vi "Configure.vi"(8 "error in (no error)":errorcluster, 11 "Measurement in":refnum<class "Measurement.lvclass">) -> (0 "error out":errorcluster, 3 "Measurement out":refnum<class "Measurement.lvclass">)   [LabVIEW 2017, in "Measurement Actor.lvlib" / "Measurement.lvclass"]
doc: "Override configure.vi to setup any parameters for a measurement before acquiring.\n\nConfigure.vi is called by the 'Initialize Measurement Actor Core.vi,' which executes before Actor Core of the root measurement class. The root configure method populates the basic Measurement UI with information such as the hardware device in use and the name of the measurement. The base configure method calls 'Acquire.vi' once execution is complete. If beginning a recurring acquisition, it reset the iteration count to zero."
uses:
  Measurement.lvclass
  C:/Program Files (x86)/National Instruments/LabVIEW 2017/vi.lib/ActorFramework/Actor/Actor.lvclass
  <vilib>/ActorFramework/Actor/Actor.lvclass/Actor.ctl
  <vilib>/ActorFramework/Message Enqueuer/Message Enqueuer.lvclass/Message Enqueuer.ctl
  Hardware/Hardware.lvclass/Hardware.ctl
  <vilib>/ActorFramework/Message Enqueuer/Init from Existing Queue.vi
  <vilib>/ActorFramework/Message Enqueuer/Enqueue.vi
  Messages/Acquire Msg/Acquire Msg.lvclass
  C:/Program Files (x86)/National Instruments/LabVIEW 2017/vi.lib/ActorFramework/Message/Message.lvclass
  <vilib>/Utility/LVClass/Get LV Class Path.vi
  <userlib>/_OpenG.lib/file/file.llb/Strip Path Extension__ogtk.vi
  <userlib>/_OpenG.lib/file/file.llb/Strip Path Extension - String__ogtk.vi
  <vilib>/ActorFramework/Message Priority Queue/Priority Enqueue.vi
  <vilib>/ActorFramework/Message Enqueuer/Message Enqueuer.lvclass
  Hardware/Hardware.lvclass
  <vilib>/ActorFramework/Actor/Actor.lvclass
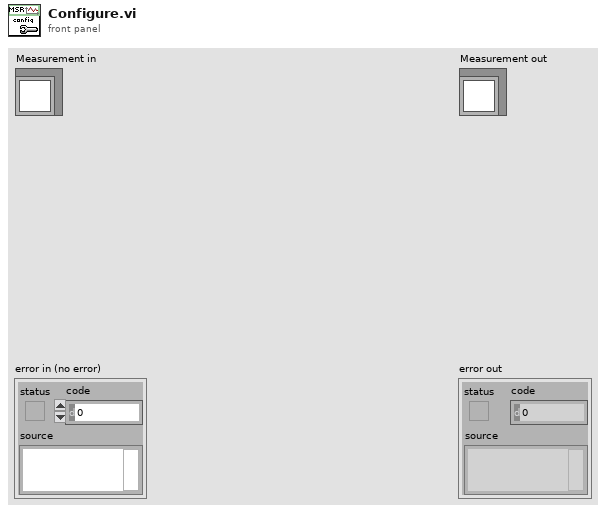
[diagram p1: front panel]
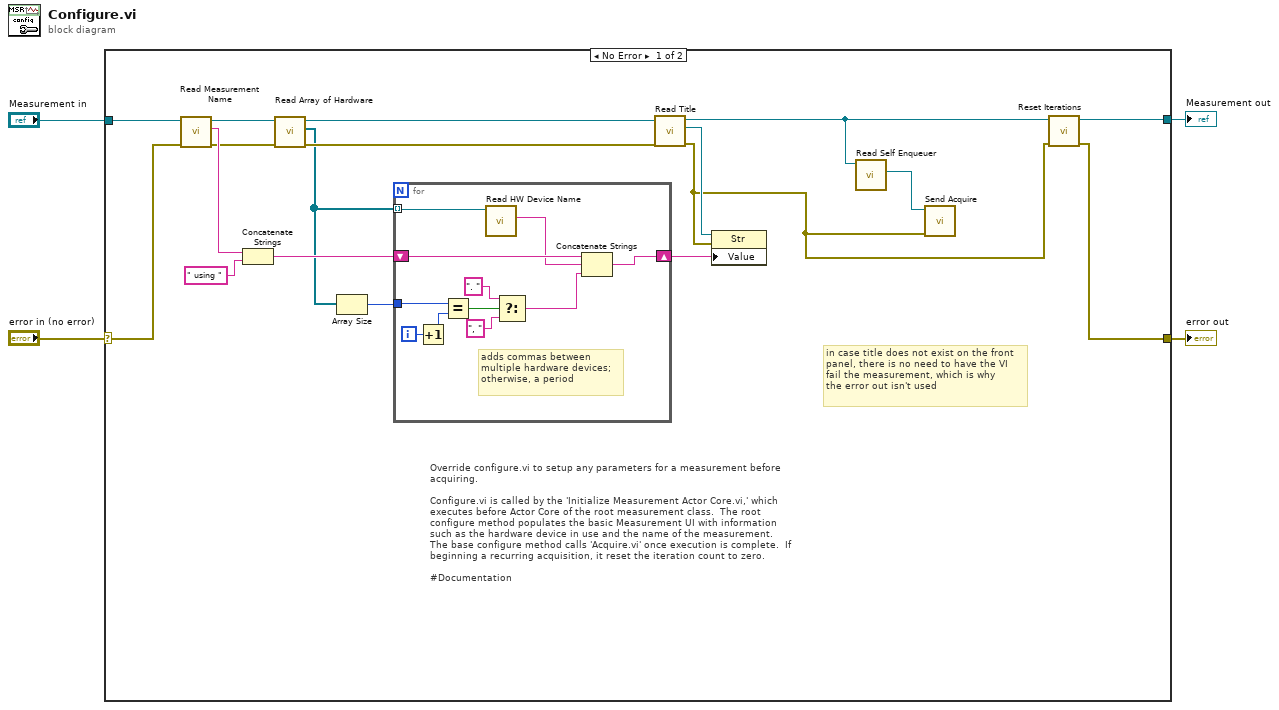
[diagram p0: block diagram]
diagram:
  n1 = case shown="No Error" "error in (no error)" {
    selector: "error in (no error)" -> [w11 w35]
    tunnel: [w8 w35] -> w3
    tunnel: [w9 w34] -> w1
    tunnel: "Measurement in" -> [w21 w34]
    frame No Error {
      # "Override configure.vi to setup any parameters for a measurement before acquiring.\n\nConfigure.vi is called by the 'Initialize Measurement Actor Core.vi,' which executes before Actor Core of the root measurement class.  The root configure method populates the basic Measurement UI with information such as the hardware device in use and the name of the measurement.  The base configure method calls 'Acquire.vi' once execution is complete.  If beginning a recurring acquisition, it reset the iteration count to zero.\n\n#Documentation"
      # "in case title does not exist on the front\npanel, there is no need to have the VI\nfail the measurement, which is why\nthe error out isn't used"
      n2 = call "Read Measurement Name.vi"("error in (no error)"=w11, "Measurement in"=w21) -> ("error out"=w13:errorcluster, "Measurement Name"=w16:string, "Measurement out"=w20:refnum<class "Measurement.lvclass">)  [unwired: 7 in]
      n3 = Concatenate Strings(w16, " using " ("string")) -> (w15:string)
      n4 = call "Read Array of Hardware.vi"("error in (no error)"=w13, "Measurement in"=w20) -> ("error out"=w12:errorcluster, "Array of Hardware"=w7:refnum<class "Hardware.lvclass">[], "Measurement out"=w19:refnum<class "Measurement.lvclass">)  [unwired: 7 in]
      n5 = Array Size(array=w7) -> (size(s)=w6:i32)
      n6 = for {
        tunnel: w7 -> [w33] mode=indexing
        shift-right: [w32] -> w18
        shift-left: w15 -> [w31]
        tunnel: w6 -> [w27]
        i -> [w29]
        # "adds commas between\nmultiple hardware devices;\notherwise, a period"
        n7 = Increment(x=w29) -> (x+1=w28:i32)
        n8 = Equal?(x=w27, y=w28) -> (x = y?=w26:bool)
        n9 = call "Read HW Device Name.vi"("Analog in"=w33) -> ("Device Name"=w30:string)  [unwired: 8 in, 2 out]
        n10 = Select(t=". " ("string"), s=w26, f=", " ("string")) -> (s? t:f=w25:string)
        n11 = Concatenate Strings(w31, w30, w25) -> (w32:string)
      }
      n12 = call "Read Title.vi"("error in (no error)"=w12, "Measurement in"=w19) -> ("error out"=w5:errorcluster, "Title"=w22:refnum<vi>, "Measurement out"=w10:refnum<class "Measurement.lvclass">)  [unwired: 7 in]
      n13 = property class="Str"(reference=w22, error in=w5, "Value"=w18) -> ()  [unwired: 2 out]
      n14 = call <vilib>:"Read Self Enqueuer.vi"("Actor"=w10) -> ("Self Enqueuer"=w14:refnum<class "Message Enqueuer.lvclass">)  [unwired: 10 in]
      n15 = call "Send Acquire.vi"("error in (no error)"=w5, "Message Enqueuer in"=w14) -> ()  [unwired: 8 in, 2 out]
      n16 = call "Reset Iterations.vi"("error in (no error)"=w5, "Measurement in"=w10) -> ("error out"=w8:errorcluster, "Measurement out"=w9:refnum<class "Measurement.lvclass">)  [unwired: 8 in]
    }
    frame Error {
    }
  }
  "error out" <- w3
  "Measurement out" <- w1
